vi "Check Available Programators.vi"(8 "error in":errorcluster, 11 "6.25":bool) -> (0 "error out":errorcluster, 1 "Tools Available":bool, 3 "standard output":string)   [LabVIEW 2023]
panel:
  out "return code":i32
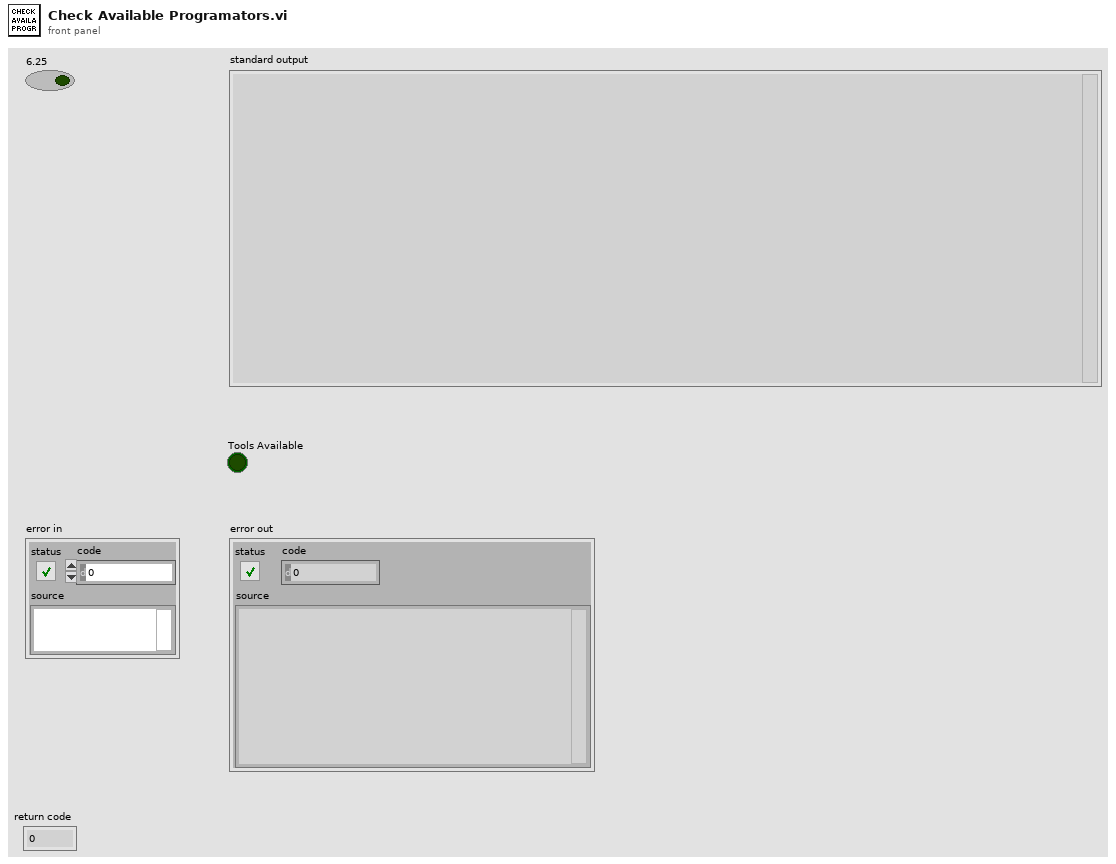
[diagram p1: front panel]
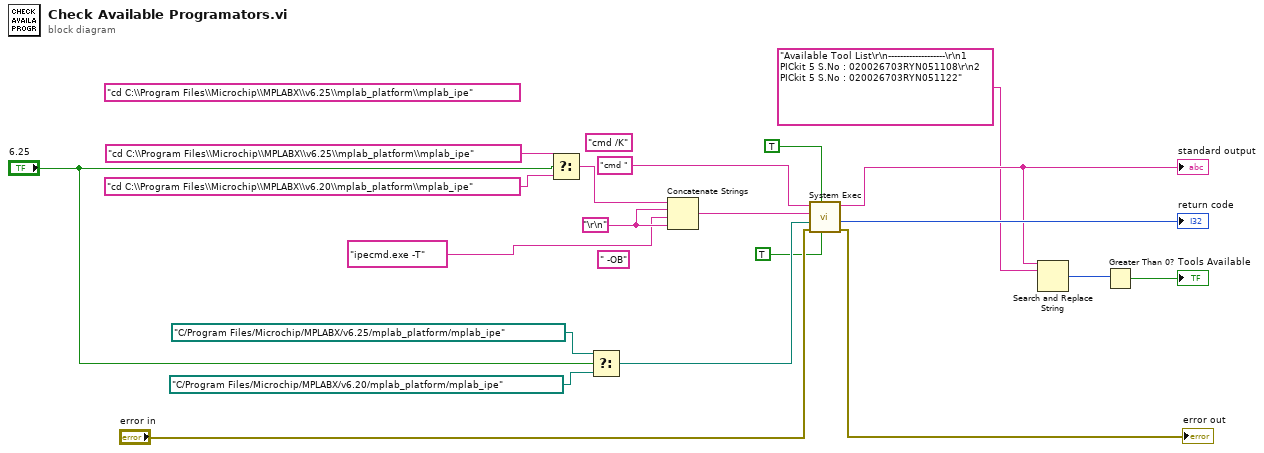
[diagram p0: block diagram]
diagram:
  (unwired) "cd C:\\Program Files\\Microchip\\MPLABX\\v6.25\\mplab_platform\\mplab_ipe" ("command line")
  (unwired) "cmd /K" ("command line")
  (unwired) " -OB" ("string")
  w11 = "\r\n"
  n1 = Select(t="cd C:\\Program Files\\Microchip\\MPLABX\\v6.25\\mplab_platform\\mplab_ipe" ("command line"), s="6.25", f="cd C:\\Program Files\\Microchip\\MPLABX\\v6.20\\mplab_platform\\mplab_ipe" ("command line")) -> (s? t:f=w6:string)
  n2 = Select(t=path "C:/Program Files/Microchip/MPLABX/v6.25/mplab_platform/mplab_ipe" ("working directory"), s="6.25", f=path "C:/Program Files/Microchip/MPLABX/v6.20/mplab_platform/mplab_ipe" ("working directory")) -> (s? t:f=w2:path)
  n3 = Concatenate Strings(w6, w11, "ipecmd.exe -T" ("command line"), w11) -> (w18:string)
  n4 = call <vilib>:"System Exec.vi"("run minimized? (F)"=TRUE, "wait until completion? (T)"=TRUE, "error in (no error)"="error in", "working directory"=w2, "standard input"=w18, "command line"="cmd ") -> ("error out"=→"error out":errorcluster, "return code"=→"return code":i32, "standard output"=w15:string)  [unwired: 2 in, 1 out]
  "standard output" <- w15
  n5 = Search and Replace String(input string=w15, search string="Available Tool List\r\n-------------------\r\n1  PICkit 5 S.No : 020026703RYN051108\r\n2  PICkit 5 S.No : 020026703RYN051122" ("standard output 2")) -> (number of replacements=w14:i32)  [unwired: 6 in, 3 out]
  n6 = Greater Than 0?(x=w14) -> (x > 0?=→"Tools Available":bool)
